vi "FPGA_DMA_Init_v1.vi"(8 "error in (no error)":errorcluster, 11 "Refnum in":T1) -> (0 "error out":errorcluster, 3 "Refnum out":T1, 5 "Remaining":u32)   [LabVIEW 2015, in "7976R_v1.lvclass"]
uses:
  <userlib>/SE-APP-Receiver/NI5772/7976R_v1/7976R_v1.lvclass
  <userlib>/SE-APP-Receiver/NI5772/7976R_v1/Private/FPGA VI Reference_DDC_v1.8.ctl
  <vilib>/rvi/interface/common/niFpgaWaitOnOcc.vi
  <vilib>/Utility/error.llb/Error Cluster From Error Code.vi
  <vilib>/rvi/errors/niLvFpgaAdjustHostInterfaceError.vi
  <vilib>/rvi/interface/nirviMethod/nirviMethod.xnode
  <vilib>/rvi/errors/niLvFpgaMergeErrorWithErrorCode.vi
  <vilib>/FPGAPlugInAG/Dynamic/niLvFpga_ReadFifo_Dynamic.vi
  <vilib>/FPGAPlugInAG/Dynamic/niLvFpga_ConfigureFifo_Dynamic.vi
  <vilib>/FPGAPlugInAG/Dynamic/niLvFpga_StartFifo_Dynamic.vi
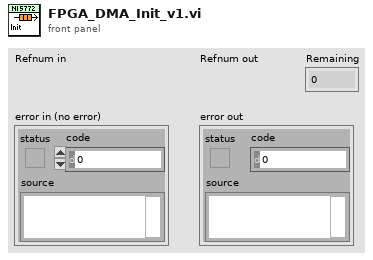
[diagram p1: front panel]
types:
  T1 = typedef "7976R_v1.lvclass/FPGA VI Reference_DDC_v1.8.ctl" = refnum<k20>
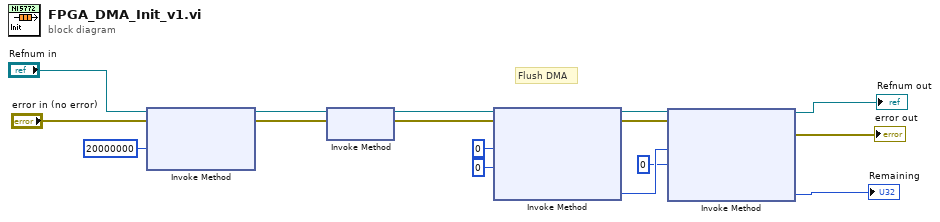
[diagram p0: block diagram]
diagram:
  # "Flush DMA"
  n1 = xnode "Invoke Method"("FPGA VI Reference In"="Refnum in", "error in"="error in (no error)", "Requested Depth"=u32 20000000 ("Depth")) -> ("FPGA VI Reference Out"=w12:T1, "error out"=w13:errorcluster)  [unwired: 1 out]
  n2 = xnode "Invoke Method"("FPGA VI Reference In"=w12, "error in"=w13) -> ("FPGA VI Reference Out"=w4:T1, "error out"=w5:errorcluster)
  n3 = xnode "Invoke Method"("FPGA VI Reference In"=w4, "error in"=w5, "Number of Elements"=u32 0, "Timeout (ms)"=0) -> ("FPGA VI Reference Out"=w7:T1, "error out"=w6:errorcluster, "Elements Remaining"=w9:u32)  [unwired: 1 out]
  n4 = xnode "Invoke Method"("FPGA VI Reference In"=w7, "error in"=w6, "Number of Elements"=w9, "Timeout (ms)"=0) -> ("FPGA VI Reference Out"=→"Refnum out":T1, "error out"=→"error out":errorcluster, "Elements Remaining"=→"Remaining":u32)  [unwired: 1 out]
